vi "WrapStrToFitButtonSize.vi"(0 "String in":string) -> (14 "Wrapped String":string)   [LabVIEW 2012, in "NEVSTOP QD Shortcuts.lvlib"]
uses:
  NEVSTOP QD Shortcuts.lvlib
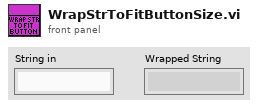
[diagram p1: front panel]
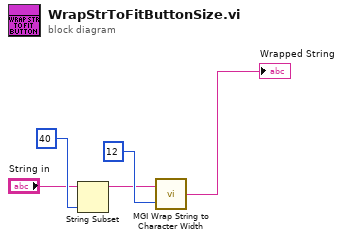
[diagram p0: block diagram]
diagram:
  n1 = String Subset(string="String in", length (rest)=40 ("length (rest)")) -> (substring=w3:string)  [unwired: 1 in]
  n2 = call <userlib>:"MGI Wrap String to Character Width.vi"("Wrap length(Characters)"=12, "Unwrapped string"=w3) -> ("Wrapped String"=→"Wrapped String":string)
